vi "Reset_Token.vi"(8 "error in (no error)":errorcluster caption="entrée d'erreur (pas d'erreur)", 10 "Reset":bool, 11 "Firebase (Default) en entrée":refnum<class "Firebase Driver.lvclass">) -> (0 "error out":errorcluster caption="sortie d'erreur", 3 "Firebase (Default) en sortie":refnum<class "Firebase Driver.lvclass">)   [LabVIEW 2020, in "Library Instrument & Equipement.lvlib" / "Library FireBase.lvlib" / "Firebase Driver.lvclass"]
uses:
  Firebase Driver.lvclass
  Firebase Driver.lvclass/Firebase Driver.ctl
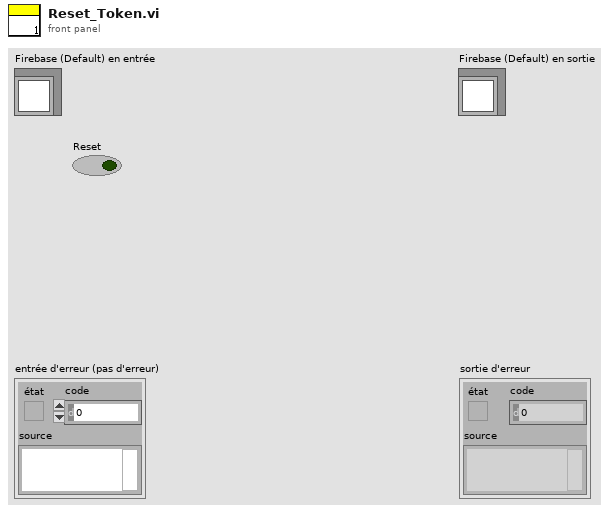
[diagram p1: front panel]
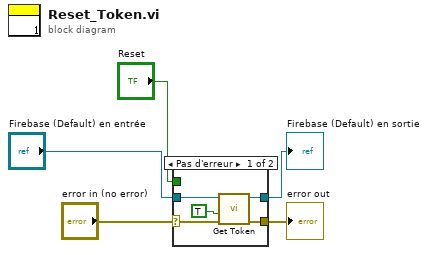
[diagram p0: block diagram]
diagram:
  n1 = case shown="Pas d'erreur" "error in (no error)" {
    selector: "error in (no error)" -> [w9 w12]
    tunnel: [w10 w12] -> w4
    tunnel: [w7 w11] -> w2
    tunnel: "Firebase (Default) en entrée" -> [w8 w11]
    tunnel: "Reset" -> [_ _]
    frame No Error {
      n2 = call-dynamic "Get Token.vi"("error in (no error)"=w9, "Reset"=TRUE, "Build Library FireBase.lvlib:Firebase (Default) IN"=w8) -> ("error out"=w10:errorcluster, "Build Library FireBase.lvlib:Firebase (Default) Out"=w7:refnum<class "Firebase Driver.lvclass">)  [unwired: 6 in, 1 out]
    }
    frame Error {
    }
  }
  "error out" <- w4
  "Firebase (Default) en sortie" <- w2
